vi "Setup Power Supply Chain.vi"(0 "reference in":refnum<class "Power Supply.lvclass">, 1 "VISA Resource Name":refnum<visa-resource-name>="Serial-Hub-1", 2 "Baud Rate":u16(ring)=3 items=["1200", "2400", "4800", "9600", "19200"], 3 "Number of Power Supplies in Chain":u8=6, 5 "error in (no error)":errorcluster) -> (14 "reference out":refnum<class "Power Supply.lvclass">, 19 "error out":errorcluster)   [LabVIEW 2017]
uses:
  Power Supply.lvclass
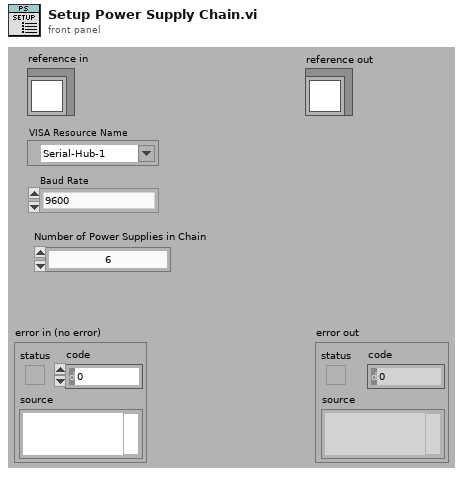
[diagram p1: front panel]
types:
  T1 = typedef "Power Supply.lvclass/ObjectAttributes.ctl" = cluster{"Power Supply Chain VISA Session":refnum<visa-resource-name>, "Power Supply Chain Address":i16, "Power Supply Open/Close Status":bool, "Power Supply Voltage Setting":dbl, "Power Supply Current Setting":dbl, "Power Supply Voltage Reading":dbl, "Power Supply Current Reading":dbl, "Power Supply Status":T2, "Power Supply Error":T3, "Fault Register":u8, "Power Supply Error":bool}
  T2 = typedef "Power Supply.lvclass/Power Supply Status.ctl" = enum16{"Closed", "Open"}
  T3 = typedef "Power Supply.lvclass/Power Supply Error.ctl" = enum16{"None", "Read Error"}
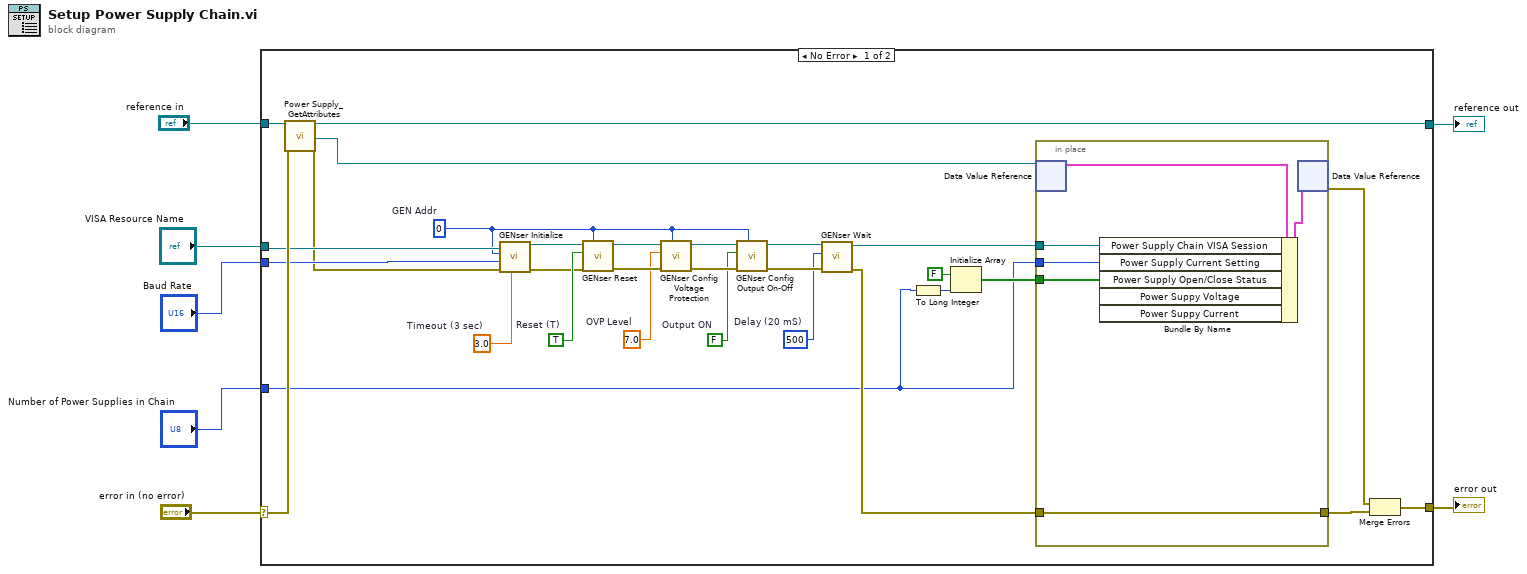
[diagram p0: block diagram]
diagram:
  n1 = case shown="No Error" "error in (no error)" {
    selector: "error in (no error)" -> [w36 w45]
    tunnel: [w33 w45] -> w6
    tunnel: [w34 w44] -> w4
    tunnel: "reference in" -> [w37 w44]
    tunnel: "Baud Rate" -> [w30 _]
    tunnel: "VISA Resource Name" -> [w29 _]
    tunnel: "Number of Power Supplies in Chain" -> [w8 _]
    frame No Error {
      w12 = u32 500  # Delay (20 mS)
      w15 = FALSE  # Output ON
      w16 = 7.0  # OVP Level
      w17 = i16 0  # GEN Addr
      w25 = TRUE  # Reset (T)
      w27 = 3.0  # Timeout (3 sec)
      n2 = call "Power Supply_GetAttributes.vi"("reference in"=w37, "error in (no error)"=w36) -> ("reference out"=w34:refnum<class "Power Supply.lvclass">, "DataRef"=w32:refnum<data-value>, "error out"=w28:errorcluster)  [unwired: 14 in, 1 out]
      n3 = call <instrlib>:"GENser Initialize.vi"("Timeout (3 sec)"=w27, "error in (no error)"=w28, "BAUD"=w30, "GEN Addr"=w17, "VISA name"=w29) -> ("error out"=w24:errorcluster, "VISA out"=w26:refnum<visa-resource-name>)  [unwired: 5 in]
      n4 = call <instrlib>:"GENser Reset.vi"("GEN Addr"=w17, "error"=w24, "Reset (T)"=w25, "VISA"=w26) -> ("error out"=w20:errorcluster, "VISA out"=w21:refnum<visa-resource-name>)  [unwired: 6 in]
      n5 = call <instrlib>:"GENser Config Voltage Protection.vi"("GEN Addr"=w17, "error"=w20, "OVP Level"=w16, "VISA"=w21) -> ("error out"=w18:errorcluster, "VISA out"=w19:refnum<visa-resource-name>)  [unwired: 6 in]
      n6 = call <instrlib>:"GENser Config Output On-Off.vi"("GEN Addr"=w17, "error"=w18, "Output ON"=w15, "VISA"=w19) -> ("error out"=w13:errorcluster, "VISA out"=w14:refnum<visa-resource-name>)  [unwired: 6 in]
      n7 = call <instrlib>:"GENser Wait.vi"("error"=w13, "Delay (20 mS)"=w12, "VISA"=w14) -> ("error out"=w10:errorcluster, "VISA out"=w11:refnum<visa-resource-name>)  [unwired: 7 in]
      n8 = To Long Integer(number=w8) -> (32bit integer=w9:i32)
      n9 = Initialize Array(FALSE, w9) -> (w22:bool[])
      n10 = in-place {
        in-place-border: w10 -> [w41]
        in-place-border: [w41] -> w31
        in-place-border: w11 -> [w40]
        in-place-border: w8 -> [w39]
        in-place-border: w22 -> [w38]
        n11 = in-place-dvr #1(w32) -> (w42:T1)  [unwired: 1 out]
        n12 = Bundle By Name(cluster=w42, "Power Supply Chain VISA Session"=w40, "Power Supply Current Setting"=w39, "Power Supply Open/Close Status"=w38) -> (w43:T1)  [unwired: 2 in]
        n13 = in-place-dvr #1(w43) -> (w35:errorcluster)  [unwired: 1 out]
      }
      n14 = Merge Errors(w35, w31) -> (w33:errorcluster)
    }
    frame Error {
    }
  }
  "error out" <- w6
  "reference out" <- w4
